vi "generate_error.vi"(6 "show_call_chain":bool=TRUE, 8 "error in (no error)":errorcluster, 10 "data":variant, 11 "error":T1) -> (0 "error out":errorcluster)   [LabVIEW 2015, in "lv-unit-conversion.lvlib"]
doc: "generate_error can be used to consistently re-create errors internally generated by the lv-unit-conversion library."
uses:
  lv-unit-conversion.lvlib
  _controls/error.ctl
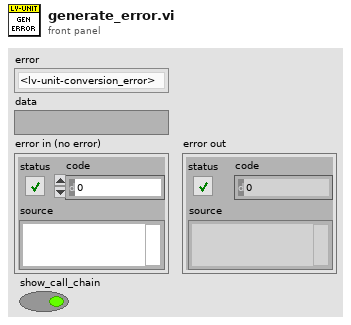
[diagram p1: front panel]
types:
  T1 = typedef "lv-unit-conversion.lvlib/error.ctl" = enum16{"<lv-unit-conversion_error>", "unit_not_found", "xml_parser", "<null>"}
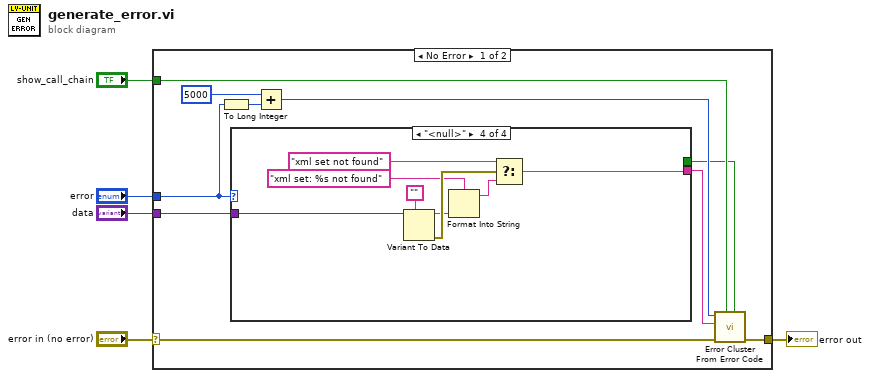
[diagram p0: block diagram]
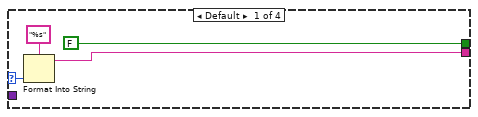
[diagram p2: hidden frame]
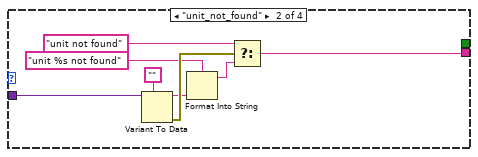
[diagram p3: hidden frame]
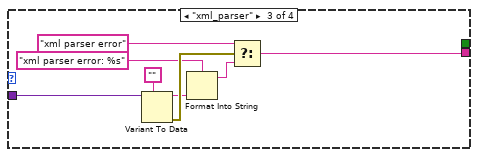
[diagram p4: hidden frame]
diagram:
  n1 = case shown="No Error" "error in (no error)" {
    selector: "error in (no error)" -> [w6 w44]
    tunnel: "data" -> [w15 _]
    tunnel: [w14 w44] -> w3
    tunnel: "error" -> [w12 _]
    tunnel: "show_call_chain" -> [w8 _]
    frame No Error {
      n2 = To Long Integer(number=w12) -> (32bit integer=w11:i32)
      n3 = case shown="\"<null>\"" w12 {
        selector: w12 -> [w18 _ _ _]
        tunnel: w15 -> [_ w26 w34 w42]
        tunnel: [w17 w22 w30 w38] -> w9
        tunnel: [FALSE _ _ _] -> w7
        frame Default {
          n4 = Format Into String(format string="%s", w18) -> (resulting string=w17:string)  [unwired: 2 in, 1 out]
        }
        frame "unit_not_found" {
          n5 = Variant To Data(type="", Variant=w26) -> (data=w21:string, error out=w27:errorcluster)  [unwired: 1 in]
          n6 = Format Into String(format string="unit %s not found", w21) -> (resulting string=w23:string)  [unwired: 2 in, 1 out]
          n7 = Select(t="unit not found" ("format string"), s=w27, f=w23) -> (s? t:f=w22:string)
        }
        frame "xml_parser" {
          n8 = Variant To Data(type="", Variant=w34) -> (data=w29:string, error out=w35:errorcluster)  [unwired: 1 in]
          n9 = Format Into String(format string="xml parser error: %s", w29) -> (resulting string=w31:string)  [unwired: 2 in, 1 out]
          n10 = Select(t="xml parser error" ("format string"), s=w35, f=w31) -> (s? t:f=w30:string)
        }
        frame "<null>" {
          n11 = Variant To Data(type="", Variant=w42) -> (data=w37:string, error out=w43:errorcluster)  [unwired: 1 in]
          n12 = Format Into String(format string="xml set: %s not found", w37) -> (resulting string=w39:string)  [unwired: 2 in, 1 out]
          n13 = Select(t="xml set not found" ("format string"), s=w43, f=w39) -> (s? t:f=w38:string)
        }
      }
      n14 = Add(x=5000, y=w11) -> (x+y=w10:i32)
      n15 = call <vilib>:"Error Cluster From Error Code.vi"("is warning? (False)"=w7, "show call chain? (False)"=w8, "error in (no error)"=w6, "error message (\"\")"=w9, "error code (0)"=w10) -> ("error out"=w14:errorcluster)  [unwired: 4 in]
    }
    frame Error {
    }
  }
  "error out" <- w3
